vi "Request Data.vi"(6 "Qualifier":string, 8 "error in (no error)":errorcluster, 9 "notifier":refnum<notifier>, 10 "Data to Send":string, 11 "Instruments in":refnum<class "Instruments.lvclass">) -> (0 "error out":errorcluster, 3 "Instruments out":refnum<class "Instruments.lvclass">)   [LabVIEW 2023, in "Instruments.lvlib" / "Instruments.lvclass"]
doc: "<b>Request Data</b>\nThis is the automation hook to Request Data from any ancestor instrument:\n\n<b>Inputs<b>\nString <b>Data to Send</b> General Request string, defined by the ancestor classes\nVariant Noitifier<b>notifier</b> This is the notifier used to control sequencing by the automation tool (ie response data is pushed into the notifier when the data is ready)\nString <b>Qualifier</b> Specific request string (example may be request measured as data to send, and channel 1 as a qualifier, resulting in a return of only channel 1 measurement data)"
uses:
  Library/Instruments.lvclass
  Library/Instruments.lvclass/Instruments.ctl
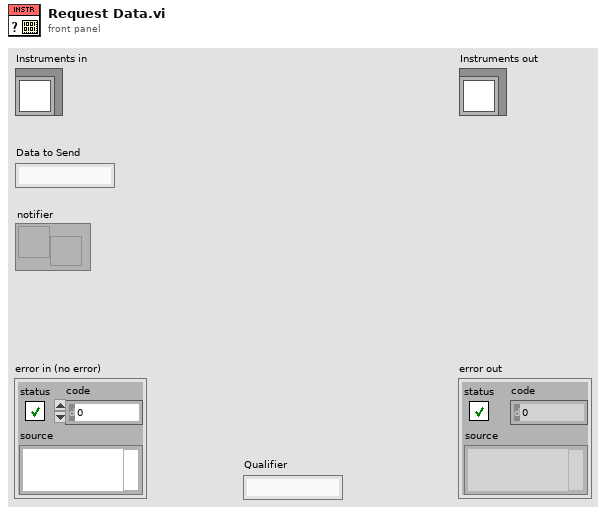
[diagram p1: front panel]
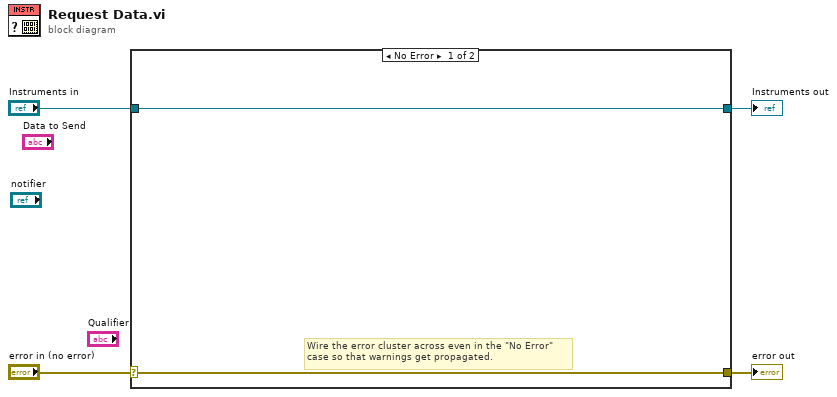
[diagram p0: block diagram]
diagram:
  n1 = case shown="No Error" "error in (no error)" {
    selector: "error in (no error)" -> [w5 w8]
    tunnel: [w5 w8] -> w3
    tunnel: [w6 w7] -> w1
    tunnel: "Instruments in" -> [w6 w7]
    frame No Error {
      # "Wire the error cluster across even in the \"No Error\"\ncase so that warnings get propagated."
    }
    frame Error {
    }
  }
  "error out" <- w3
  "Instruments out" <- w1
